vi "random array opg 4.1.vi"() -> ()   [LabVIEW 2015]
panel:
  in  "# of elements":i32
  in  "Start Subset":i32
  in  "Scaling Factor":dbl
  out "Final Array":dbl[](array[numeric])
  out "Subset array":dbl[](array[numeric])
  out "Random Array":dbl[](array[numeric])
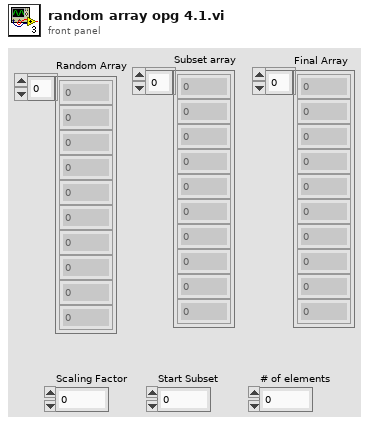
[diagram p1: front panel]
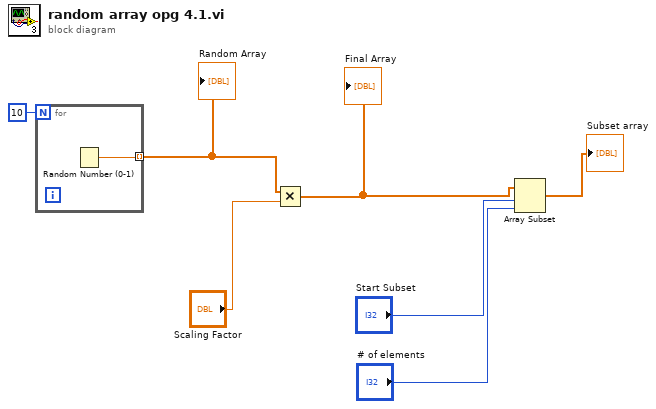
[diagram p0: block diagram]
diagram:
  n1 = for {
    N: 10 -> [_]
    tunnel: [w8] -> w5 mode=indexing
    n2 = Random Number (0-1)() -> (number: 0 to 1=w8:dbl)
  }
  "Random Array" <- w5
  n3 = Multiply(x=w5, y="Scaling Factor") -> (x*y=w1:dbl[])
  "Final Array" <- w1
  n4 = Array Subset(array=w1, index="Start Subset", length="# of elements") -> (→"Subset array":dbl[])
